vi "Broadcast Event.vi"(8 "error in (no error)":errorcluster, 9 "Event Data":refnum<class "Event.lvclass">, 10 "View Enqueuer":refnum<class "Message Enqueuer.lvclass">, 11 "Controller in":refnum<class "Controller.lvclass">) -> (0 "error out":errorcluster, 3 "Controller out":refnum<class "Controller.lvclass">)   [LabVIEW 2023, in "MVC Actors.lvlib" / "Controller.lvclass"]
uses:
  Controller.lvclass
  Event/Event.lvclass
  <vilib>/ActorFramework/Message Enqueuer/Message Enqueuer.lvclass
  Controller.lvclass/Controller.ctl
  Event Handler Details.ctl
  Event Handlers/Abstract Event Message for View/Abstract Event Message for View.lvclass
  C:/Program Files/National Instruments/LabVIEW 2023/vi.lib/ActorFramework/Message/Message.lvclass
  Event Handlers/Abstract Event Message for View/Abstract Event Message for View.lvclass/Abstract Event Message for View.ctl
  <vilib>/ActorFramework/Message Enqueuer/Message Enqueuer.lvclass/Message Enqueuer.ctl
  <vilib>/ActorFramework/Message Enqueuer/Enqueue.vi
  <vilib>/Utility/LVClass/Get LV Class Name.vi
  <resource>/AFDebug/Generate Trace for Message.vi
  <vilib>/ActorFramework/Message Priority Queue/Priority Enqueue.vi
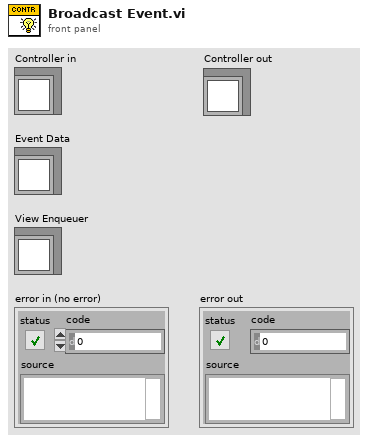
[diagram p1: front panel]
types:
  T1 = typedef "MVC Actors.lvlib/Controller.lvclass/Event Handler Details.ctl" = cluster{"Exclude From Broadcast":bool, "Paused":bool, "View Event Fire Handler":refnum<class "Abstract Event Message for View.lvclass">}
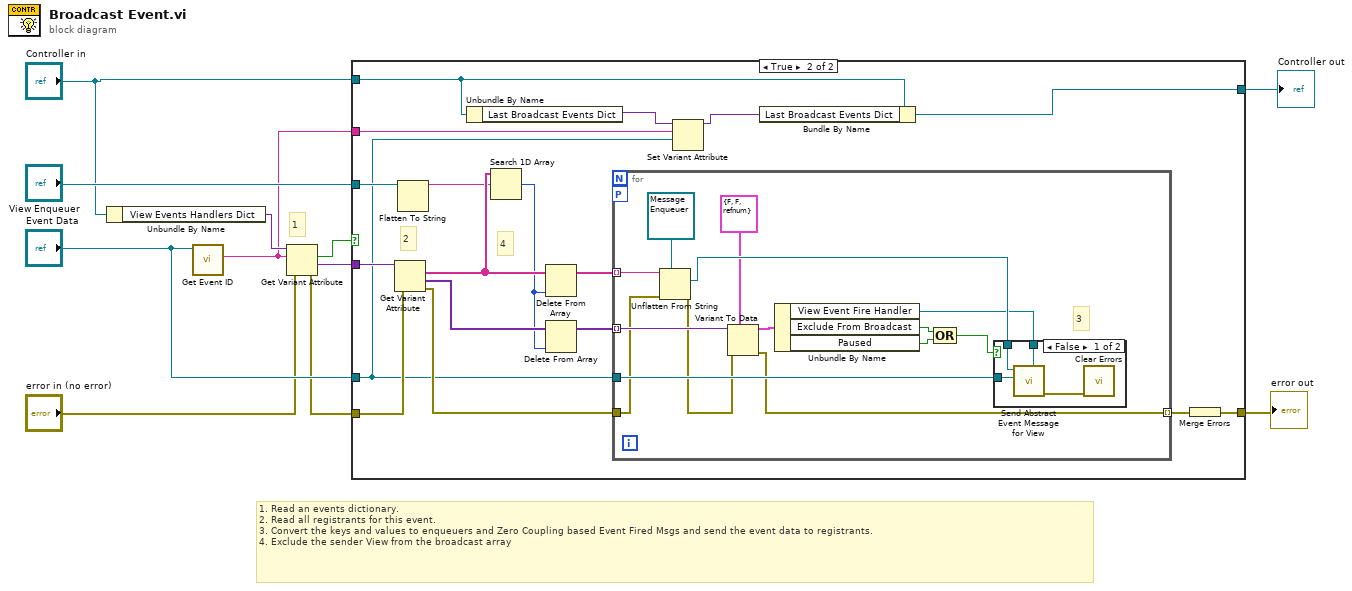
[diagram p0: block diagram]
diagram:
  # "1. Read an events dictionary.\n2. Read all registrants for this event.\n3. Convert the keys and values to enqueuers and Zero Coupling based Event Fired Msgs and send the event data to registrants.\n4. Exclude the sender View from the broadcast array"
  # "1"
  n1 = Unbundle By Name("Controller in") -> ("View Events Handlers Dict"=w4:variant)
  n2 = call-dynamic "Get Event ID.vi"("Event in"="Event Data") -> ("Event ID"=w2:string)  [unwired: 8 in, 2 out]
  n3 = Get Variant Attribute(Variant=w4, name=w2, error in="error in (no error)") -> (found=w7:bool, value=w6:variant, error out=w5:errorcluster)  [unwired: 1 in, 1 out]
  n4 = case shown="True" w7 {
    tunnel: w6 -> [_ w30]
    tunnel: "Event Data" -> [_ w15]
    tunnel: w5 -> [w13 w29]
    tunnel: [w13 w20] -> w10
    tunnel: "View Enqueuer" -> [_ w25]
    tunnel: "Controller in" -> [w12 w17]
    tunnel: w2 -> [_ w16]
    tunnel: [w12 w14] -> w1
    frame False {
    }
    frame True {
      # "4"
      # "2"
      n5 = Get Variant Attribute(Variant=w30, error in=w29) -> (names=w27:string[], values=w23:variant[], error out=w28:errorcluster)  [unwired: 2 in, 1 out]
      n6 = Flatten To String(anything=w25) -> (data string=w24:string)  [unwired: 3 in, 2 out]
      n7 = Unbundle By Name(w17) -> ("Last Broadcast Events Dict"=w19:variant)
      n8 = Search 1D Array(1D array=w27, element=w24) -> (index of element=w21:i32)  [unwired: 1 in]
      n9 = Delete From Array(array=w27, index=w21) -> (array with subset deleted=w26:string[])  [unwired: 1 in, 1 out]
      n10 = Delete From Array(array=w23, index=w21) -> (array with subset deleted=w22:variant[])  [unwired: 1 in, 1 out]
      n11 = for {
        tunnel: w26 -> [w45] mode=indexing
        tunnel: w22 -> [w44] mode=indexing
        tunnel: w15 -> [w41]
        tunnel: w28 -> [w40]
        tunnel: [w36] -> w31 mode=indexing
        workers-P: _ -> [_]
        # "3"
        n12 = Unflatten From String(type=refnum<class "Message Enqueuer.lvclass"> refnum ("Message Enqueuer"), binary string=w45, error in (no error)=w40) -> (value=w43:refnum<class "Message Enqueuer.lvclass">, error out=w39:errorcluster)  [unwired: 2 in, 1 out]
        n13 = Variant To Data(error in=w39, type=T1 {"Exclude From Broadcast"=FALSE, "Paused"=FALSE, "View Event Fire Handler"=refnum} ("Message Type"), Variant=w44) -> (data=w42:T1, error out=w36:errorcluster)
        n14 = Unbundle By Name(w42) -> ("View Event Fire Handler"=w34:refnum<class "Abstract Event Message for View.lvclass">, "Exclude From Broadcast"=w33:bool, "Paused"=w32:bool)
        n15 = Compound Arithmetic op=OR(w33, w32) -> (w35:bool)
        n16 = case shown="False" w35 {
          tunnel: w34 -> [w49 _]
          tunnel: w41 -> [w48 _]
          tunnel: w43 -> [w46 _]
          frame False {
            n17 = call "Send Abstract Event Message for View.vi"("Message Type"=w49, "Event Data"=w48, "Message Enqueuer"=w46) -> ("Error Out"=w47:errorcluster)  [unwired: 7 in, 1 out]
            n18 = call <vilib>:"Clear Errors.vi"("error in (no error)"=w47) -> ()  [unwired: 5 in, 2 out]
          }
          frame True {
          }
        }
      }
      n19 = Set Variant Attribute(Variant=w19, name=w16, value=w15) -> (Variant out=w18:variant)  [unwired: 1 in, 2 out]
      n20 = Bundle By Name(cluster=w17, "Last Broadcast Events Dict"=w18) -> (w14:refnum<class "Controller.lvclass">)
      n21 = Merge Errors(w31) -> (w20:errorcluster)
    }
  }
  "error out" <- w10
  "Controller out" <- w1
